vi "Eth Status Write Inputs.vi"(7 "Status Reference":T1, 8 "error in (no error)":errorcluster, 9 "Write Enable":bool[](array[boolean]), 10 "Start":bool[](array[boolean]), 11 "Lenght":i32) -> (0 "error out":errorcluster, 5 "Status Reference out":T1)   [LabVIEW 2019, in "Eth Status.lvlib"]
uses:
  Eth Status.lvlib
  Ctl/Status.ctl
  MB_TCP2/MB_TCP_State.ctl
  MB_TCP2/MB_TCP.lvclass
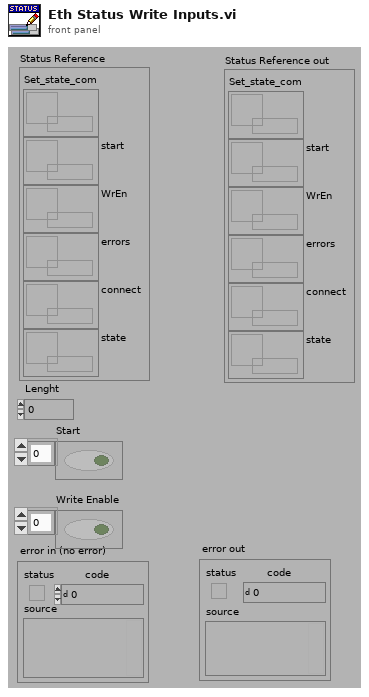
[diagram p1: front panel]
types:
  T1 = typedef "Eth Status.lvlib/Status.ctl" = cluster{"Set_state_com":refnum<data-value>, "start":refnum<data-value>, "WrEn":refnum<data-value>, "errors":refnum<data-value>, "connect":refnum<data-value>, "state":refnum<data-value>}
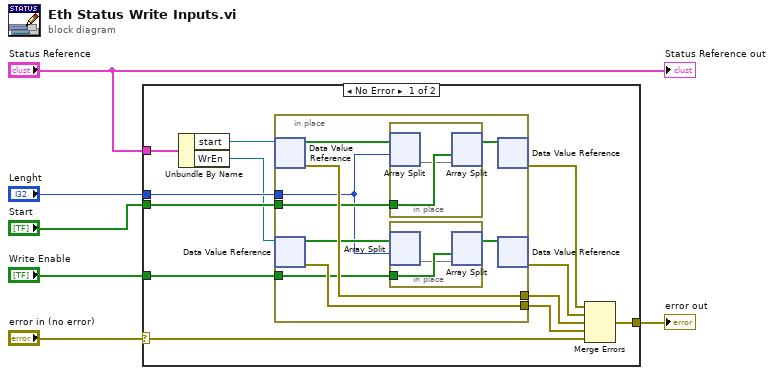
[diagram p0: block diagram]
diagram:
  n1 = case shown="No Error" "error in (no error)" {
    selector: "error in (no error)" -> [w7 w32]
    tunnel: [w16 w32] -> w5
    tunnel: "Lenght" -> [w18 _]
    tunnel: "Status Reference" -> [w17 _]
    tunnel: "Start" -> [w15 _]
    tunnel: "Write Enable" -> [w13 _]
    frame No Error {
      n2 = Unbundle By Name(w17) -> ("start"=w9:refnum<data-value>, "WrEn"=w8:refnum<data-value>)
      n3 = in-place {
        in-place-border: w18 -> [w19]
        in-place-border: [w27] -> w14
        in-place-border: w15 -> [w25]
        in-place-border: w13 -> [w21]
        in-place-border: [w23] -> w10
        n4 = in-place-dvr #1(w9) -> (w26:bool[], w27:errorcluster)
        n5 = in-place-dvr #2(w8) -> (w22:bool[], w23:errorcluster)
        n6 = in-place {
          in-place-border: w25 -> [w31]
          n7 = in-place-split #3(w26, w19) -> (w30:bool[])  [unwired: 1 out]
          n8 = in-place-split #3(w31, w30) -> (w24:bool[])  [unwired: 1 out]
        }
        n9 = in-place {
          in-place-border: w21 -> [w29]
          n10 = in-place-split #4(w22, w19) -> (w28:bool[])  [unwired: 1 out]
          n11 = in-place-split #4(w29, w28) -> (w20:bool[])  [unwired: 1 out]
        }
        n12 = in-place-dvr #1(w24) -> (w12:errorcluster)  [unwired: 1 out]
        n13 = in-place-dvr #2(w20) -> (w11:errorcluster)  [unwired: 1 out]
      }
      n14 = Merge Errors(w12, w11, w14, w10, w7) -> (w16:errorcluster)
    }
    frame Error {
    }
  }
  "error out" <- w5
  "Status Reference out" <- "Status Reference"
